vi "Get External Time.vi"(8 "error in (no error)":errorcluster, 10 "ClockID":u8, 11 "Clock Convert Map in":T1) -> (0 "error out":errorcluster, 1 "T0":i64, 2 "Time (ns)":i64, 3 "Clock Convert Map out":T1)   [LabVIEW 2021, in "Time_CIF_U.lvlib"]
doc: "This will determine an external clock based on the system time and the correlation points provided by the Clock Conversion Map. This allows the system to track and accurately convert multiple different clocks on the system. This is useful for systems with multiple external clocks (multi-DUT testing, multiple external time sources, etc)."
uses:
  Time_CIF_U.lvlib
  Typedef/Clock Conversion Map.ctl
  Typedef/Timestamp Pair.ctl
  SubVIs/Add Error.vi
  System Time/LabVIEW Time to TAI Time.vi
  Errors/Append Error Location.vi
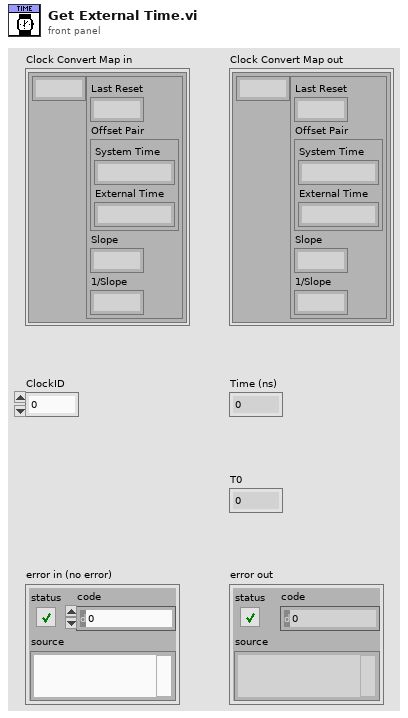
[diagram p1: front panel]
types:
  T1 = typedef "Time_CIF_U.lvlib/Clock Conversion Map.ctl" = map{u8, cluster{"Last Reset":i64, "Offset Pair":T2, "Slope":dbl, "1/Slope":dbl}}
  T2 = typedef "Time_CIF_U.lvlib/Timestamp Pair.ctl" = cluster{"System Time":i64, "External Time":i64}
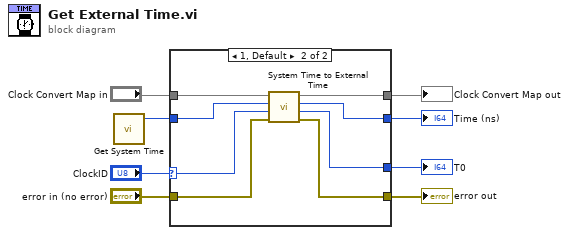
[diagram p0: block diagram]
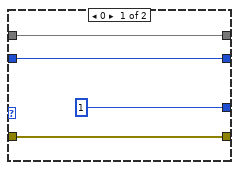
[diagram p2: hidden frame]
diagram:
  n1 = call "Get System Time.vi"() -> ("Time (ns)"=w3:i64)  [unwired: 5 in]
  n2 = case shown="1, Default" "ClockID" {
    selector: "ClockID" -> [_ w17]
    tunnel: [w10 w16] -> w8
    tunnel: "error in (no error)" -> [w12 w14]
    tunnel: [w12 w13] -> w5
    tunnel: [i64 1 ("UTC Time (ns)") w15] -> w4
    tunnel: w3 -> [w10 w18]
    tunnel: "Clock Convert Map in" -> [w9 w20]
    tunnel: [w9 w19] -> w1
    frame 0 {
    }
    frame 1, Default {
      n3 = call "System Time to External Time.vi"("error in (no error)"=w14, "ClockID"=w17, "System Time"=w18, "Clock Convert Map in"=w20) -> ("error out"=w13:errorcluster, "Last Reset Time"=w15:i64, "External Time"=w16:i64, "Clock Convert Map out"=w19:T1)  [unwired: 4 in]
    }
  }
  "error out" <- w5
  "Time (ns)" <- w8
  "T0" <- w4
  "Clock Convert Map out" <- w1
